vi "CM-TDT-Save Device.vi"(0 "configuration file path":path=path "C:/PXI Connections.txt", 7 "Device":T1, 11 "error in (no error)":errorcluster) -> (15 "error out":errorcluster)   [LabVIEW 2020]
uses:
  PXI DAQ VIs/TDT VIs/Typedefs/TDT-Device Config.ctl
  PXI DAQ VIs/TDT VIs/Typedefs/TDT-Output source.ctl
  PXI DAQ VIs/TDT VIs/Typedefs/TDT-Device ID.ctl
  PXI DAQ VIs/TDT VIs/Typedefs/TDT-Input source.ctl
  <vilib>/Utility/config.llb/Write Key (String).vi
  <vilib>/Utility/config.llb/Write Key (I32).vi
  <vilib>/Utility/config.llb/NI_LVConfig.lvlib
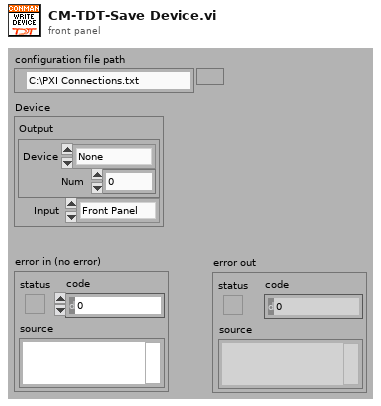
[diagram p1: front panel]
types:
  T1 = typedef "TDT-Device Config.ctl" = cluster{"Output":T2, "Input":T4}
  T2 = typedef "TDT-Output source.ctl" = cluster{"Device":T3, "Num":i32}
  T3 = typedef "TDT-Device ID.ctl" = enum16{"None", "PA5", "RP2", "RL2", "RA16", "RV8", "RX5", "RX6", "RX7", "RX8", "RZ2", "RZ5", "RZ6"}
  T4 = typedef "TDT-Input source.ctl" = enum16{"Front Panel", "RA4LI", "RA16LI"}
  T5 = typedef "NI_LVConfig.lvlib/Config Data RefNum.ctl" = refnum<k1>
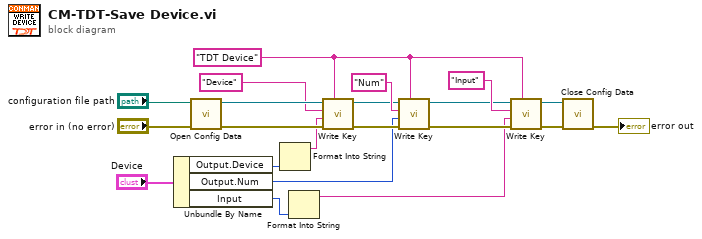
[diagram p0: block diagram]
diagram:
  w15 = "TDT Device" ("section")
  n1 = Unbundle By Name("Device") -> ("Output.Device"=w16:T3, "Output.Num"=w3:i32, "Input"=w2:T4)
  n2 = call <vilib>:"Open Config Data.vi"("error in (no error)"="error in (no error)", "configuration file path"="configuration file path") -> ("error out"=w17:errorcluster, "refnum"=w18:T5)  [unwired: 7 in, 1 out]
  n3 = Format Into String(w16) -> (resulting string=w5:string)  [unwired: 3 in, 1 out]
  n4 = Format Into String(w2) -> (resulting string=w1:string)  [unwired: 3 in, 1 out]
  n5 = call-poly <vilib>:"Write Key.vi"("section"=w15, "error in (no error)"=w17, "value"=w5, "key"="Device", "refnum"=w18) -> ("error out"=w10:errorcluster, "refnum out"=w9:T5)  [unwired: 4 in, 1 out]
  n6 = call-poly <vilib>:"Write Key.vi"("section"=w15, "error in (no error)"=w10, "value"=w3, "key"="Num", "refnum"=w9) -> ("error out"=w13:errorcluster, "refnum out"=w12:T5)  [unwired: 4 in, 1 out]
  n7 = call-poly <vilib>:"Write Key.vi"("section"=w15, "error in (no error)"=w13, "value"=w1, "key"="Input", "refnum"=w12) -> ("error out"=w6:errorcluster, "refnum out"=w7:T5)  [unwired: 4 in, 1 out]
  n8 = call <vilib>:"Close Config Data.vi"("error in (no error)"=w6, "refnum"=w7) -> ("error out"=→"error out":errorcluster)  [unwired: 8 in, 1 out]
